vi "SRV_Error 56 Dialog.vi"(7 "SRV In":refnum<k5>, 8 "error in (no error)":errorcluster, 9 "In Pico":bool, 11 "Control Queue":refnum<queue>) -> (0 "error out":errorcluster, 1 "Retry?":bool, 3 "Control Queue out":refnum<queue>, 5 "SRV Out":refnum<k5>)   [LabVIEW 2014]
doc: "This VI is not generally useful for Error 56 error handling. It is specifically designed for the \"Init TCP\" case of MainController VI only.\n\n\nAuthor: Mike Schultz"
uses:
  Support/SRV_Command-Data Queue Data Type.ctl
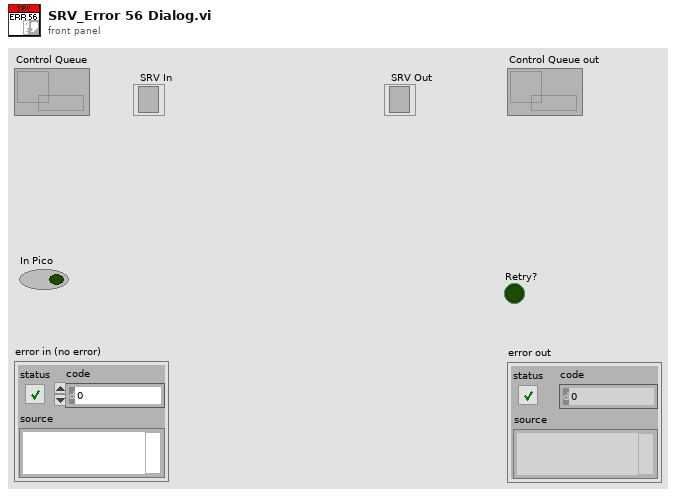
[diagram p1: front panel]
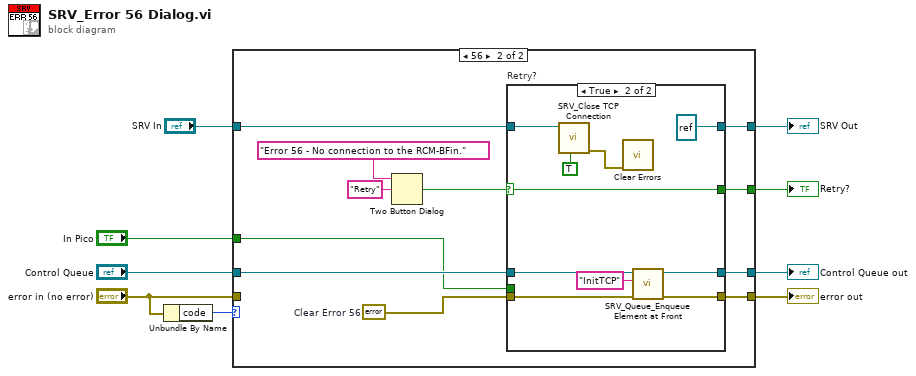
[diagram p0: block diagram]
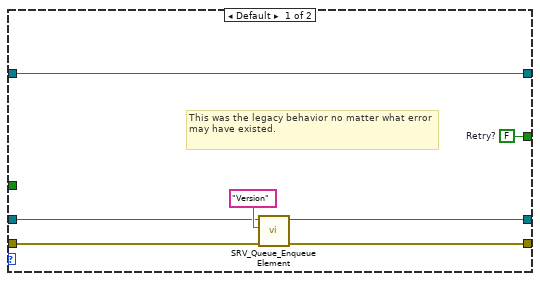
[diagram p2: hidden frame]
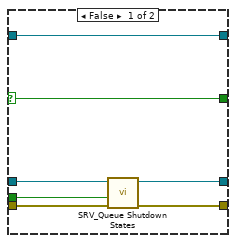
[diagram p3: hidden frame]
diagram:
  n1 = Unbundle By Name("error in (no error)") -> ("code"=w7:i32)
  n2 = case shown="56" w7 {
    tunnel: "error in (no error)" -> [w13 _]
    tunnel: [w12 w24] -> w9
    tunnel: "Control Queue" -> [w15 w23]
    tunnel: [w14 w22] -> w5
    tunnel: "In Pico" -> [_ w21]
    tunnel: "SRV In" -> [w11 w19]
    tunnel: [w11 w18] -> w2
    tunnel: [w10 w17] -> w1
    frame Default {
      w10 = FALSE  # Retry?
      # "This was the legacy behavior no matter what error may have existed."
      n3 = call "SRV_Queue_Enqueue Element.vi"("error in (no error)"=w13, "Command"="Version" ("element"), "Command-Data Queue"=w15) -> ("error out"=w12:errorcluster, "Command-Data Queue out"=w14:refnum<queue>)  [unwired: 6 in, 1 out]
    }
    frame 56 {
      w20 = errorcluster {"status"=FALSE, "code"=0, "source"=""}  # Clear Error 56
      n4 = Two Button Dialog(message="Error 56 - No connection to the RCM-BFin.", 2:"Retry" ("T button name (\"OK\")")) -> (T button?=w25:bool)  [unwired: 1 in]
      n5 = case "Retry?" shown="True" w25 {
        selector: w25 -> [w28 w36]
        tunnel: w20 -> [w30 w44]
        tunnel: [w34 w43] -> w24
        tunnel: w23 -> [w33 w42]
        tunnel: [w32 w41] -> w22
        tunnel: w21 -> [w31 _]
        tunnel: w19 -> [w29 w39]
        tunnel: [w29 refnum<k5> refnum ("SRV Out")] -> w18
        tunnel: [w28 w36] -> w17
        frame False {
          n6 = call "SRV_Queue Shutdown States.vi"("error in (no error)"=w30, "In Pico"=w31, "Control Queue"=w33) -> ("error out"=w34:errorcluster, "Control Queue out"=w32:refnum<queue>)  [unwired: 7 in]
        }
        frame True {
          n7 = call "SRV_Close TCP Connection.vi"("Force Reset? (F)"=TRUE, "connection ID"=w39) -> ("error out"=w38:errorcluster)  [unwired: 9 in]
          n8 = call <vilib>:"Clear Errors.vi"("error in (no error)"=w38) -> ()  [unwired: 5 in, 2 out]
          n9 = call "SRV_Queue_Enqueue Element at Front.vi"("error in (no error)"=w44, "Command"="InitTCP", "Command-Data Queue"=w42) -> ("error out"=w43:errorcluster, "Command-Data Queue out"=w41:refnum<queue>)  [unwired: 6 in, 1 out]
        }
      }
    }
  }
  "error out" <- w9
  "Control Queue out" <- w5
  "SRV Out" <- w2
  "Retry?" <- w1
